vi "Message type.vi"(11 "IHandleGoodby in":refnum<class "IHandleGoodby.lvclass">) -> (2 "Internal message type":T1, 3 "IHandleGoodby out":refnum<class "IHandleGoodby.lvclass">)   [LabVIEW 2020, in "wamplv.lvlib" / "IHandleGoodby.lvclass"]
uses:
  IHandleGoodby.lvclass
  TypeDefs/Internal message type.ctl
  wamplv.lvlib
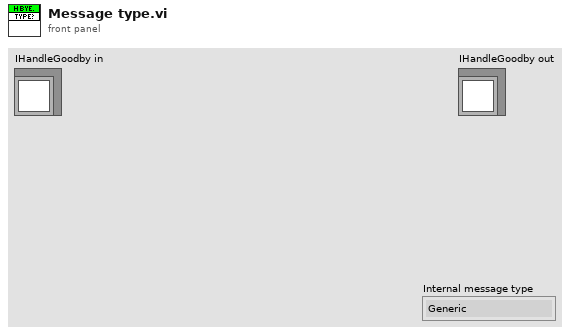
[diagram p1: front panel]
types:
  T1 = typedef "wamplv.lvlib/Internal message type.ctl" = enum16{"Generic", "Generic with write output", "Handle Result", "Handle Error", "Handle Abort", "Handle Welcome", "Handle Goodbye", "Send abort"}
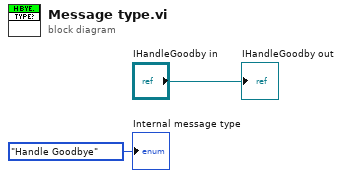
[diagram p0: block diagram]
diagram:
  "IHandleGoodby out" <- "IHandleGoodby in"
  "Internal message type" <- Internal_message_type."Handle Goodbye" ("Internal message type")
